vi "GOOP_LVClass_Item_OnRename.vi"(11 "Object":u64) -> ()   [LabVIEW 2020]
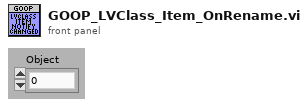
[diagram p1: front panel]
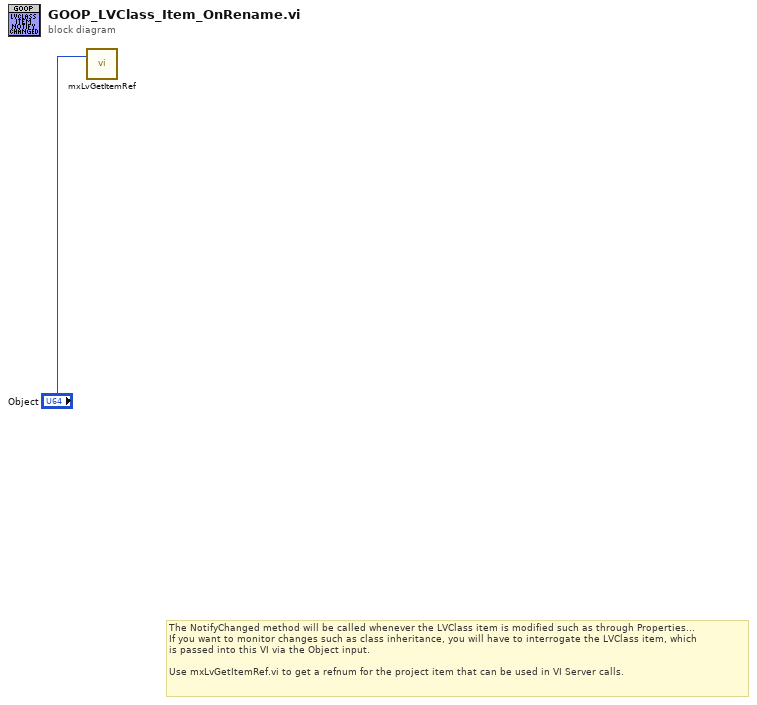
[diagram p0: block diagram]
diagram:
  # "The NotifyChanged method will be called whenever the LVClass item is modified such as through Properties...\nIf you want to monitor changes such as class inheritance, you will have to interrogate the LVClass item, which\nis passed into this VI via the Object input.\n\nUse mxLvGetItemRef.vi to get a refnum for the project item that can be used in VI Server calls."
  n1 = call <resource>:"mxLvGetItemRef.vi"("Item"="Object") -> ()  [unwired: 1 in, 3 out]
